vi "Wrist-Intake_TEST.vi"(8 "error constant":errorcluster, 11 "Cluster 2":T1) -> (0 "error constant 2":errorcluster, 3 "Cluster":T1)   [LabVIEW 2018]
uses:
  TypeDefs/Teleop Data Cluster.ctl
  TypeDefs/Joystick Axes.ctl
  TypeDefs/Joystick Buttons.ctl
panel:
  in  "wrist scale factor":dbl=0.5 format="%#_13g"
  in  "lower speed":dbl=-0.8 format="%#_13g"
  in  "upper speed":dbl=0.8 format="%#_13g"
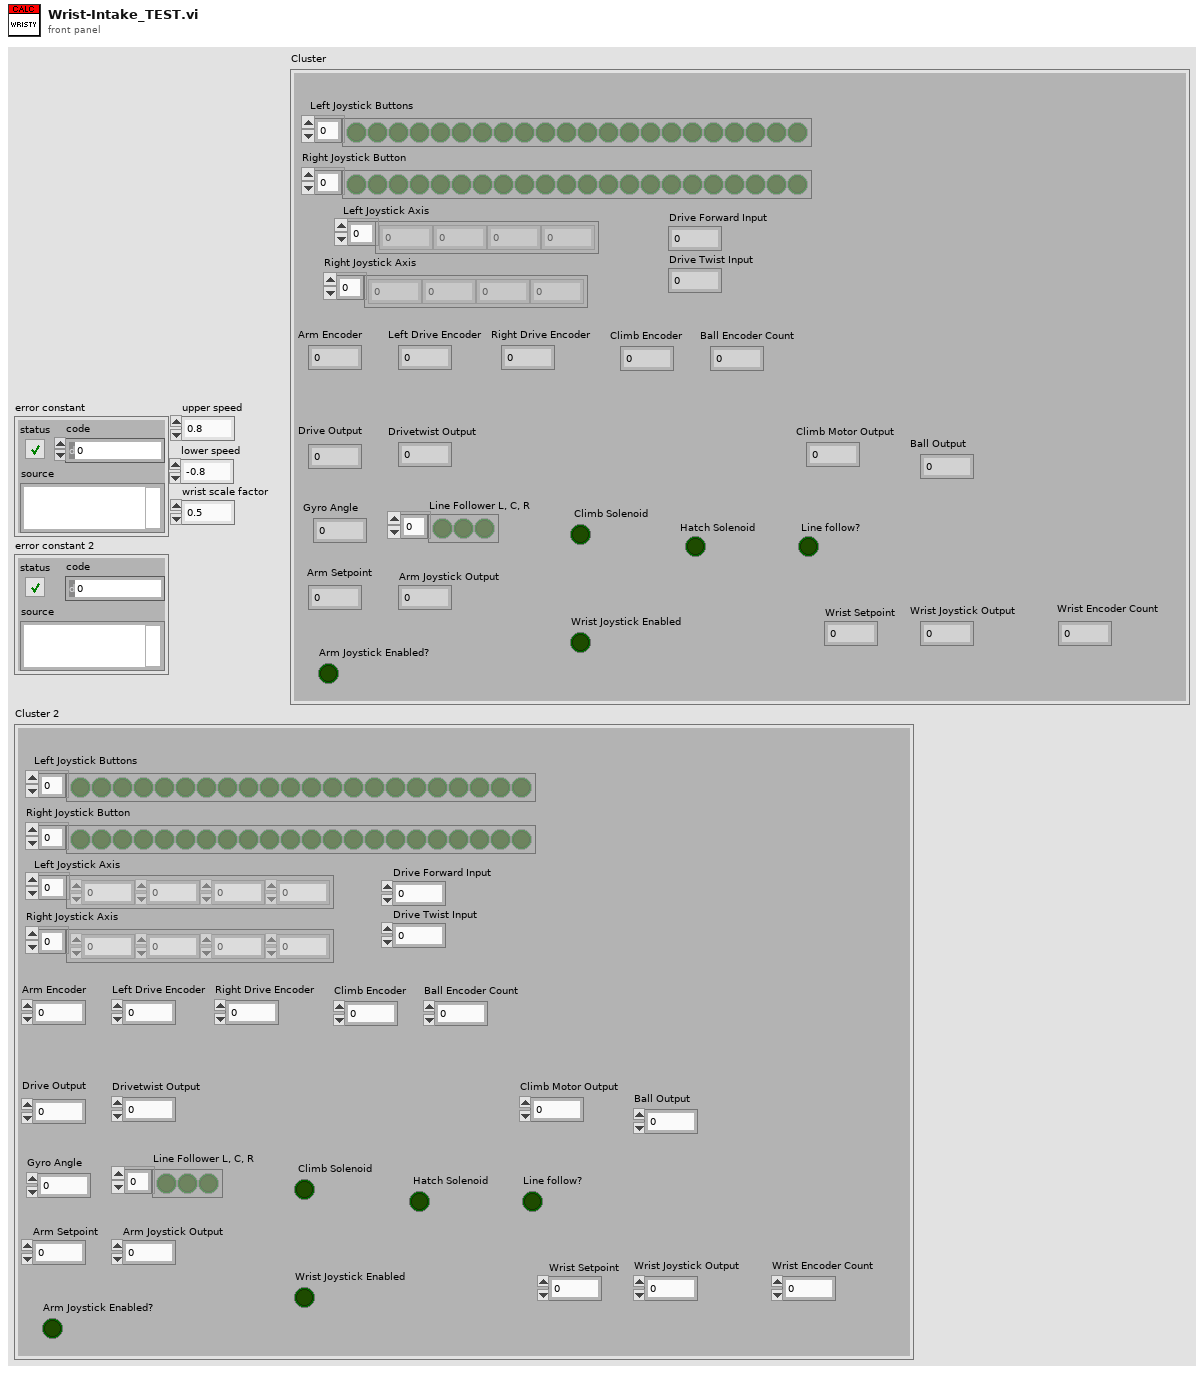
[diagram p1: front panel]
types:
  T1 = typedef "Teleop Data Cluster.ctl" = cluster{"Drive Forward Input ":dbl, "Drive Twist Input":dbl, "Drive Output":dbl, "Drivetwist Output":dbl, "Left Joystick Buttons":bool[], "Left Joystick Axis":dbl[], "Right Joystick Axis":dbl[], "Right Joystick Button":bool[], "Arm Encoder":dbl, "Left Drive Encoder":dbl, "Right Drive Encoder":dbl, "Gyro Angle ":dbl, "Arm Joystick Output  ":dbl, "Line Follower L, C, R ":bool[], "Line follow?":bool, " Climb Solenoid":bool, "Wrist Encoder Count":dbl, "Wrist Joystick Output":dbl, "Ball Encoder Count":dbl, "Ball Output":dbl, "Climb Encoder":dbl, "Climb Motor Output":dbl, " Hatch Solenoid":bool, "Arm Setpoint ":dbl, "Wrist Setpoint ":dbl, "Arm Joystick Enabled?":bool, "Wrist Joystick Enabled":bool}
  T2 = typedef "Joystick Buttons.ctl" = enum16{"Trigger", "Thumb", "Top 3", "Top 4", "Top 5", "Top 6", "Bottom 7", "Bottom 8", "Bottom 9", "Bottom 10", "Bottom 11", "Bottom 12"}
  T3 = typedef "Joystick Axes.ctl" = enum16{"X Axis", "Y Axis", "Twist Axis", "Throttle"}
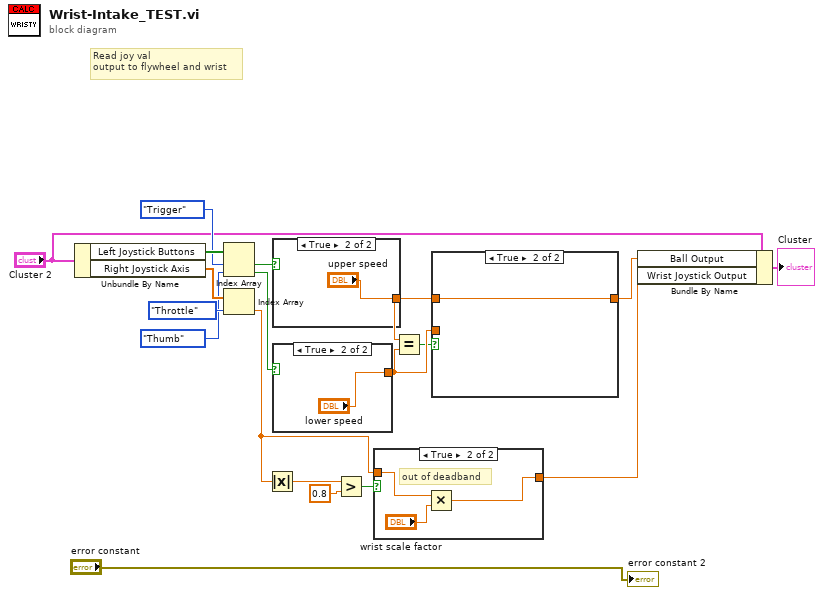
[diagram p0: block diagram]
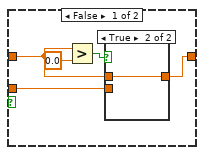
[diagram p2: hidden frame]
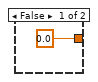
[diagram p4: hidden frame]
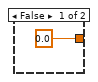
[diagram p5: hidden frame]
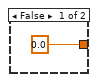
[diagram p6: hidden frame]
diagram:
  # "Read joy val\noutput to flywheel and wrist"
  n1 = Unbundle By Name("Cluster 2") -> ("Left Joystick Buttons"=w17:bool[], "Right Joystick Axis"=w19:dbl[])
  n2 = Index Array(array=w17, index #1=Joystick_Buttons."Trigger" ("Enum"), index #2=Joystick_Buttons."Thumb" ("Enum")) -> (element #1=w14:bool, element #2=w13:bool)
  n3 = Index Array(array=w19, index=Joystick_Axes."Throttle" ("Enum")) -> (element=w9:dbl)
  n4 = Absolute Value(x=w9) -> (abs(x)=w12:dbl)
  n5 = case shown="True" w14 {
    tunnel: [0.0 "upper speed"] -> w7
    frame False {
    }
    frame True {
    }
  }
  n6 = case shown="True" w13 {
    tunnel: [0.0 "lower speed"] -> w6
    frame False {
    }
    frame True {
    }
  }
  n7 = Greater?(x=w12, y=0.8) -> (0:w10:bool)
  n8 = case shown="True" w10 {
    tunnel: w9 -> [_ w26]
    tunnel: [0.0 w25] -> w4
    frame False {
    }
    frame True {
      # "out of deadband"
      n9 = Multiply(x=w26, y="wrist scale factor") -> (x*y=w25:dbl)
    }
  }
  n10 = Equal?(x=w7, y=w6) -> (x = y?=w2:bool)
  n11 = case shown="True" w2 {
    tunnel: [w29 w35] -> w8
    tunnel: w7 -> [w30 w35]
    tunnel: w6 -> [w28 _]
    frame False {
      n12 = Greater?(x=w30, y=0.0) -> (0:w31:bool)
      n13 = case shown="True" w31 {
        tunnel: w30 -> [_ w34]
        tunnel: [w33 w34] -> w29
        tunnel: w28 -> [w33 _]
        frame False {
        }
        frame True {
        }
      }
    }
    frame True {
    }
  }
  n14 = Bundle By Name(cluster="Cluster 2", "Ball Output"=w8, "Wrist Joystick Output"=w4) -> (→"Cluster":T1)
  "error constant 2" <- "error constant"
